vi "100Pic.vi"() -> ()   [LabVIEW 2016]
uses:
  <vilib>/userdefined/High Color/IMAQdx.ctl
  <vilib>/vision/Measure.llb/Edge Options.ctl
  <vilib>/vision/Measure.llb/Edge Polarity.ctl
  <vilib>/vision/driver/NI_Vision_Acquisition_Software.lvlib
  <vilib>/vision/NI_Vision_Development_Module.lvlib
panel:
  out "Prossing":i32
  out "Fitted Circle":T1 {"Average SNR (dB)" format="%.2f"; "Average Strength" format="%.2f"; "Roundness (Real-World)" format="%.2f"; "Radius (Real-World)" format="%.2f"; "Center (Real-World)"."Y" format="%.2f"; "Center (Real-World)"."X" format="%.2f"; "Radius (Pixels)" format="%.2f"; "Center (Pixels)"."Y" format="%.2f"; "Center (Pixels)"."X" format="%.2f"}
  out "Image":T2(plugin-control)
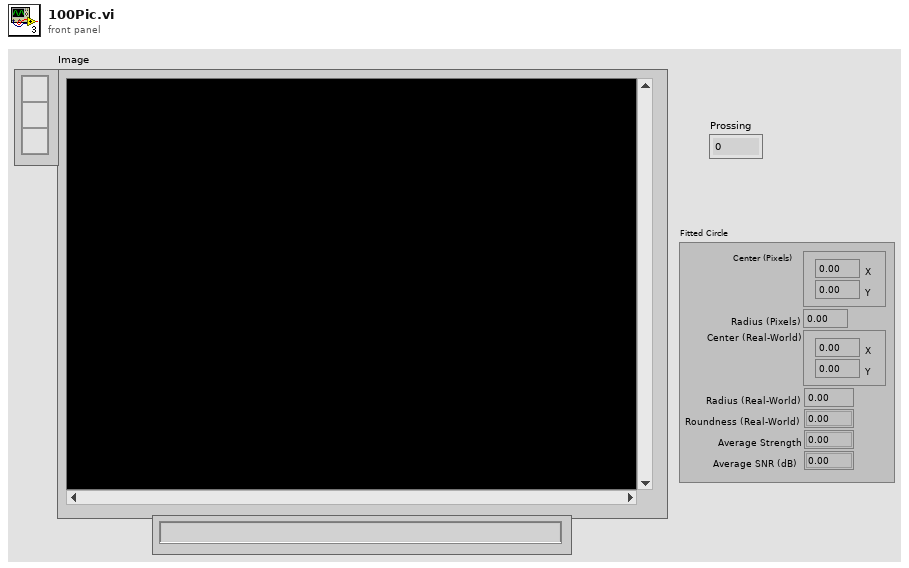
[diagram p1: front panel]
types:
  T1 = cluster{"Center (Pixels)":cluster{"X":sgl, "Y":sgl}, "Radius (Pixels)":dbl, "Center (Real-World)":cluster{"X":sgl, "Y":sgl}, "Radius (Real-World)":dbl, "Roundness (Real-World)":dbl, "Average Strength":dbl, "Average SNR (dB)":dbl}
  T2 = typedef "IMAQ Image.ctl" = refnum<image>
  T3 = typedef "IMAQdx.ctl" = refnum<k21>
  T4 = typedef "IMAQ Circle" = cluster{"Center X":i32, "Center Y":i32, "Inner Radius":i32, "Outer Radius":i32, "Start Angle":dbl, "End Angle":dbl}
  T5 = cluster{"Left":i32, "Top":i32, "Right":i32, "Bottom":i32}
  T6 = typedef "Edge Options.ctl" = cluster{"Edge Polarity":T7, "Kernel Size":u32, "Width":u32, "Minimum Edge Strength":sgl, "Interpolation Type":enum32{"Zero Order", "Bilinear", "Quadratic", "Cubic", "Bilinear Fixed"}, "Data Processing Method":enum32{"Average", "Median"}}
  T7 = typedef "Edge Polarity.ctl" = u32
  T8 = cluster{"Search  Direction":u32, "Edge Options":T6, "Show Search Area":bool, "Show Search Lines":bool, "Show Edges Found":bool, "Show Result":bool, "Search Area Color":u32, "Search Lines Color":u32, "Edge Locations Color":u32, "Result Color":u32, "Overlay Group Name":string}
  T9 = cluster{"Process":enum16{"Get First Edge", "Get First + Last Edge", "Get All Edges", "Get Best Edge"}, "Step Size":dbl, "Max Pixel Radius":i32}
  T10 = typedef "Image Type" = u32
  T11 = typedef "ROI Descriptor" = cluster{"Global Rectangle":i32[], "Contours":cluster{"ID":enum32{"External", "Internal"}, "Type":u32, "Coordinates":i32[]}[]}
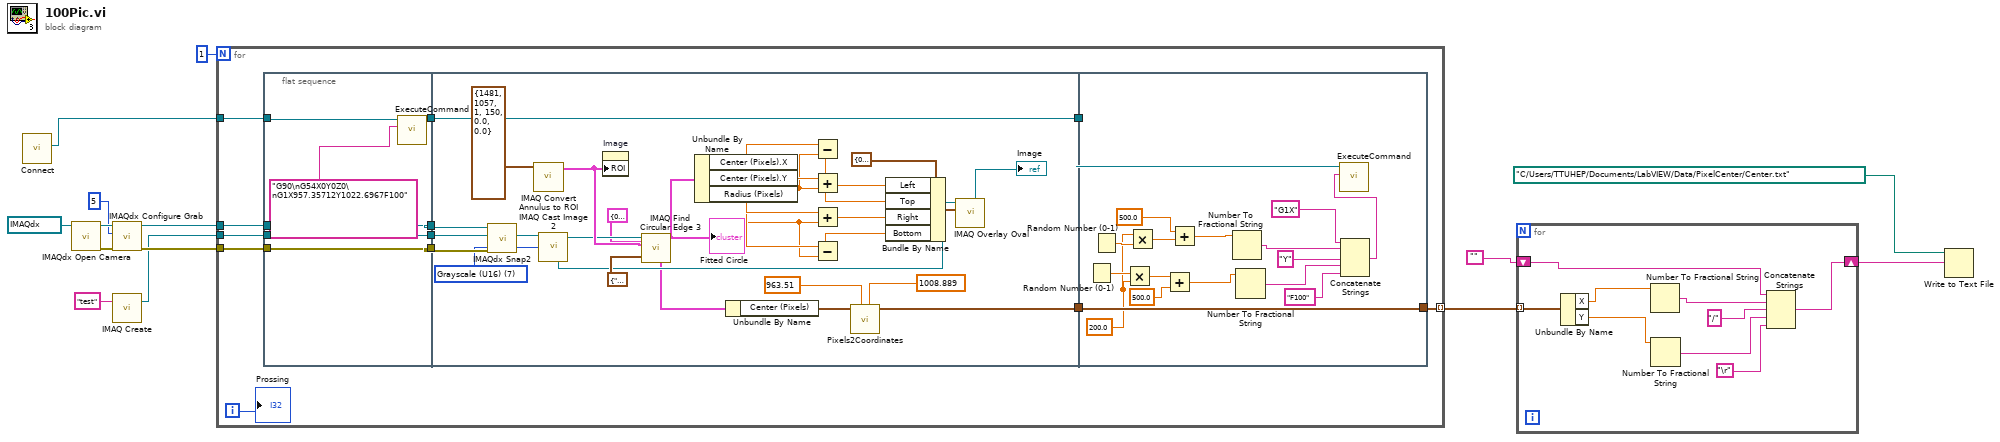
[diagram p0: block diagram]
diagram:
  n1 = call "Connect.vi"() -> ("controller"=w5:refnum<k24>)  [unwired: 10 in, 1 out]
  n2 = call <vilib>:"IMAQdx Open Camera.vi"("Session In"=T3 "cam0") -> ("error out"=w12:errorcluster, "Session Out"=w13:T3)  [unwired: 9 in]
  n3 = call <vilib>:"IMAQdx Configure Grab.vi"("error in"=w12, "Number of Buffers"=u32 5, "Session In"=w13) -> ("error out"=w9:errorcluster, "Session Out"=w10:T3)  [unwired: 7 in]
  n4 = call "IMAQ Create"("Image Name"="test") -> ("New Image"=w7:T2)  [unwired: 4 in, 1 out]
  n5 = for {
    N: 1 -> [_]
    tunnel: w10 -> [w26]
    tunnel: w9 -> [w25]
    tunnel: w7 -> [w24]
    tunnel: w5 -> [w20]
    tunnel: [w16] -> w4 mode=indexing
    i -> [w15]
    n6 = flat-sequence {
      tunnel: w24 -> [w30]
      tunnel: w25 -> [w31]
      tunnel: w26 -> [w32]
      tunnel: [w32] -> w23
      tunnel: [w31] -> w22
      tunnel: [w30] -> w21
      tunnel: w20 -> [w29]
      tunnel: [w27] -> w18
      tunnel: w23 -> [w58]
      tunnel: w22 -> [w57]
      tunnel: w21 -> [w56]
      tunnel: [w37] -> w19
      tunnel: w18 -> [w37]
      tunnel: [w35] -> w17
      tunnel: w19 -> [w75]
      tunnel: w17 -> [w74]
      tunnel: [w74] -> w16
      frame #0 {
        n7 = call "ExecuteCommand.vi"("Command Code"="G90\nG54X0Y0Z0\nG1X957.35712Y1022.6967F100", "controller in"=w29) -> ("controller out"=w27:refnum<k24>)  [unwired: 7 in, 2 out]
      }
      frame #1 {
        w55 = T10 7 items=["Grayscale (U8)", "Grayscale (I16)", "Grayscale (SGL)", "Complex (CSG)", "RGB (U32)", "HSL (U32)", "RGB (U64)", "Grayscale (U16)"] ("Image Type")
        n8 = call <vilib>:"IMAQdx Snap2.vi"("error in"=w57, "Image In"=w56, "Session In"=w58) -> ("Image Out"=w54:T2)  [unwired: 6 in, 2 out]
        n9 = call "IMAQ Convert Annulus to ROI"("Annulus"=T4 {"Center X"=1481, "Center Y"=1057, "Inner Radius"=1, "Outer Radius"=150, "Start Angle"=0.0, "End Angle"=0.0}) -> ("ROI Descriptor"=w51:T11)  [unwired: 8 in, 1 out]
        n10 = call "IMAQ Cast Image 2"("Image Src"=w54, "Image Type"=w55) -> ("Image Dst Out"=w49:T2)  [unwired: 12 in, 1 out]
        n11 = property on="Image" class="ImageControl"("ROI"=w51) -> ()  [unwired: 2 in, 2 out]
        n12 = call "IMAQ Find Circular Edge 3"("Circle Fit Options"=T9 {"Process"=enum."Get First Edge", "Step Size"=3.0, "Max Pixel Radius"=3}, "Options"=T8 {"Search  Direction"=0, "Edge Options"={"Edge Polarity"=0, "Kernel Size"=3, "Width"=3, "Minimum Edge Strength"=10.0, "Interpolation Type"=enum."Bilinear Fixed", "Data Processing Method"=enum."Average"}, "Show Search Area"=TRUE, "Show Search Lines"=FALSE, "Show Edges Found"=TRUE, "Show Result"=TRUE, "Search Area Color"=65280, "Search Lines Color"=255, "Edge Locations Color"=16776960, "Result Color"=16711680, "Overlay Group Name"=""}, "ROI Descriptor"=w51, "Image"=w49) -> ("Fitted Circle"=w38:T1)  [unwired: 3 in, 4 out]
        "Fitted Circle" <- w38
        n13 = Unbundle By Name(w38) -> ("Center (Pixels).X"=w47:sgl, "Center (Pixels).Y"=w46:sgl, "Radius (Pixels)"=w45:dbl)
        n14 = Unbundle By Name(w38) -> ("Center (Pixels)"=w36:cluster{"X":sgl, "Y":sgl})
        n15 = Subtract(x=w47, y=w45) -> (x-y=w41:dbl)
        n16 = Add(x=w46, y=w45) -> (x+y=w40:dbl)
        n17 = Add(x=w47, y=w45) -> (x+y=w42:dbl)
        n18 = Subtract(x=w46, y=w45) -> (x-y=w39:dbl)
        n19 = call "Pixels2Coordinates.vi"("Y"=1008.889, "X"=963.51, "Location (Pixel)"=w36) -> ("output cluster"=w35:cluster{"X":sgl, "Y":sgl})  [unwired: 8 in]
        n20 = Bundle By Name(cluster=T5 {"Left"=0, "Top"=0, "Right"=0, "Bottom"=0} ("Bounding Rectangle"), "Left"=w41, "Top"=w40, "Right"=w42, "Bottom"=w39) -> (w43:T5)
        n21 = call "IMAQ Overlay Oval"("Bounding Rectangle"=w43, "Image"=w49) -> ("Image Out"=→"Image":T2)  [unwired: 8 in, 1 out]
      }
      frame #2 {
        w71 = 200.0
        n22 = Random Number (0-1)() -> (number: 0 to 1=w72:dbl)
        n23 = Random Number (0-1)() -> (number: 0 to 1=w73:dbl)
        n24 = Multiply(x=w72, y=w71) -> (x*y=w69:dbl)
        n25 = Multiply(x=w71, y=w73) -> (x*y=w70:dbl)
        n26 = Add(x=w69, y=500.0) -> (x+y=w65:dbl)
        n27 = Add(x=500.0, y=w70) -> (x+y=w66:dbl)
        n28 = Number To Fractional String(number=w66) -> (F-format string=w63:string)  [unwired: 3 in]
        n29 = Number To Fractional String(number=w65) -> (F-format string=w61:string)  [unwired: 3 in]
        n30 = Concatenate Strings("G1X", w63, "Y", w61, "F100") -> (w59:string)
        n31 = call "ExecuteCommand.vi"("Command Code"=w59, "controller in"=w75) -> ()  [unwired: 7 in, 3 out]
      }
    }
    "Prossing" <- w15
  }
  n32 = for {
    tunnel: w4 -> [w84] mode=indexing
    shift-right: [w77] -> w2
    shift-left: "" -> [w76]
    n33 = Unbundle By Name(w84) -> ("X"=w83:sgl, "Y"=w82:sgl)
    n34 = Number To Fractional String(number=w83) -> (F-format string=w81:string)  [unwired: 3 in]
    n35 = Number To Fractional String(number=w82) -> (F-format string=w80:string)  [unwired: 3 in]
    n36 = Concatenate Strings(w76, w81, "/" ("string"), w80, "\r") -> (w77:string)
  }
  n37 = Write to Text File(file (use dialog)=path "C:/Users/TTUHEP/Documents/LabVIEW/Data/PixelCenter/Center.txt", text=w2) -> ()  [unwired: 2 in, 3 out]
